vi "Write DAC Settings.vi"(10 "DAC Settings":T1={"Voltage Reference"=4.096, "Min Counts"=0, "Max Counts"=65535} {"Voltage Reference" format="%.3f"}, 11 "VoltageToILCDACRaw in":refnum<class "VoltageToILCDACRaw.lvclass">) -> (3 "VoltageToILCDACRaw out":refnum<class "VoltageToILCDACRaw.lvclass">)   [LabVIEW 2015, in "VoltageToILCDACRaw.lvclass"]
uses:
  VoltageToILCDACRaw.lvclass
  Typedefs/DAC Settings.ctl
  VoltageToILCDACRaw.lvclass/VoltageToILCDACRaw.ctl
  Typedefs/FAMTTypedefs.lvlib
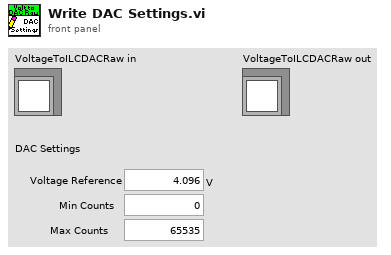
[diagram p1: front panel]
types:
  T1 = typedef "FAMTTypedefs.lvlib/DAC Settings.ctl" = cluster{"Voltage Reference":dbl[unit], "Min Counts":i32, "Max Counts":i32}
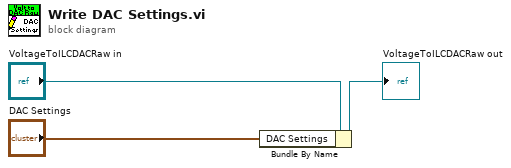
[diagram p0: block diagram]
diagram:
  n1 = Bundle By Name(cluster="VoltageToILCDACRaw in", "DAC Settings"="DAC Settings") -> (→"VoltageToILCDACRaw out":refnum<class "VoltageToILCDACRaw.lvclass">)
